vi "HIOKI PW3390 Acquisition Harmonic.vi"() -> ()   [LabVIEW 2009]
doc: "Outputs the harmonic measurement data and plots on a bar graph in 100ms cycle."
uses:
  <instrlib>/PW3390/Common/_Initialize/HIOKI PW3390 Initialize LAN.vi
  <instrlib>/PW3390/Common/_Initialize/HIOKI PW3390 Initialize RS-232C.vi
panel:
  out "error out":errorcluster
  in  "Communication Interface":enum16{"LAN", "RS-232C"}(ring)
  in  "COM Port":refnum<visa-resource-name>="COM1"
  in  "baud rate (38400bps)":u32=38400
  in  "IP Address":string="192.168.1.1"
  out "HP Phase":dbl[](graph)
  out "HI Phase":dbl[](graph)
  out "HU Phase":dbl[](graph)
  out "HP %":dbl[](graph)
  out "HI %":dbl[](graph)
  out "HU %":dbl[](graph)
  out "HU Value":dbl[](graph)
  out "HP Value":dbl[](graph)
  out "HI Value":dbl[](graph)
  out "Data out":dbl[](array[numeric])
  out "Selected Item out":string[](array[string])
  in  "Stop":bool
  in  "CH Select":T1(ring)
  # "Note:\n Please set configuration before starting the program.\nChanging configuration during running the program is invalid."
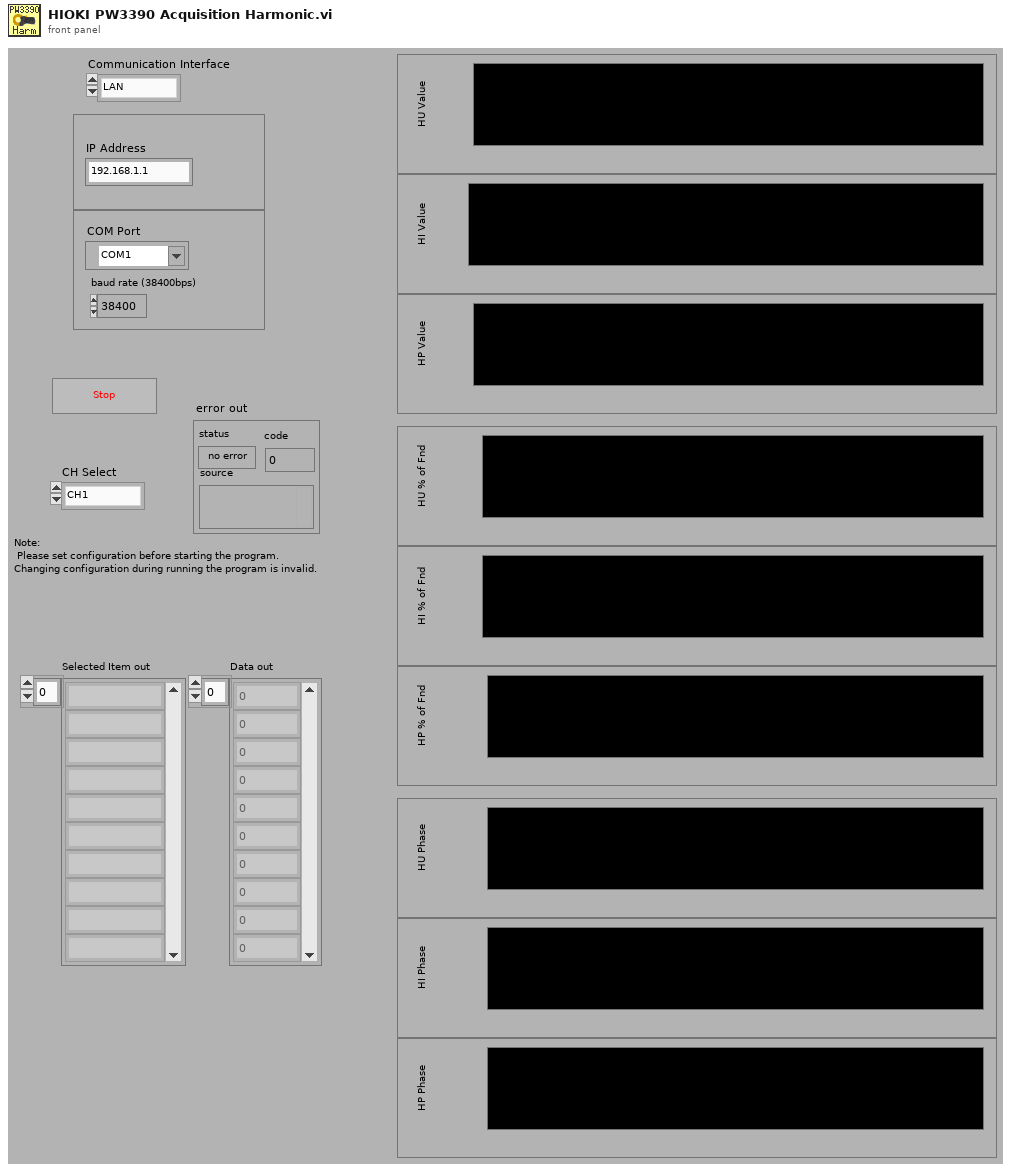
[diagram p1: front panel]
types:
  T1 = enum16{"CH1", "CH2", "CH3", "CH4", "CH12", "CH34", "CH123"}
  T2 = cluster{"LIST1":bool[], "LIST2":bool[], "LIST1 2":bool[], "LIST2 2":bool[], "LIST1 3":bool[], "LIST2 3":bool[]}
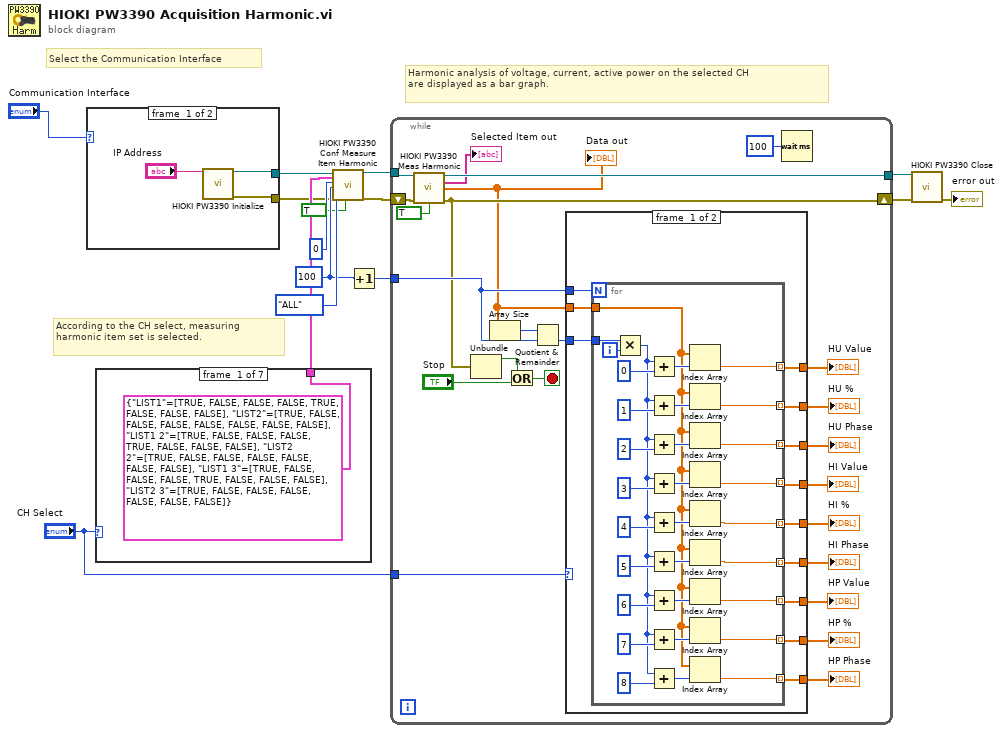
[diagram p0: block diagram]
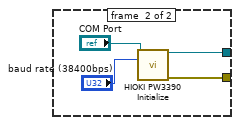
[diagram p2: hidden frame]
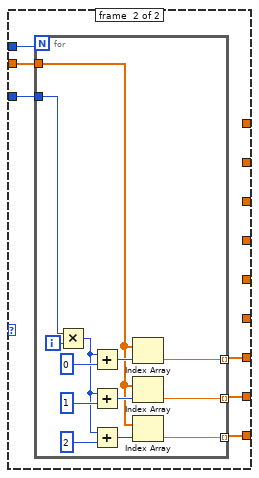
[diagram p3: hidden frame]
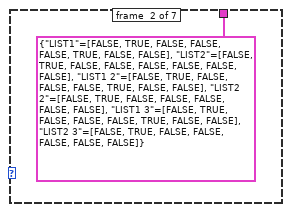
[diagram p4: hidden frame]
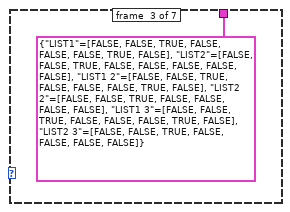
[diagram p5: hidden frame]
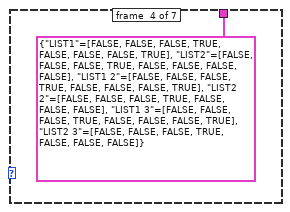
[diagram p6: hidden frame]
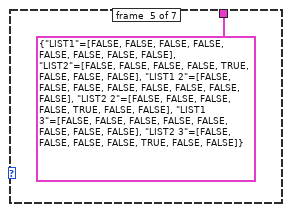
[diagram p7: hidden frame]
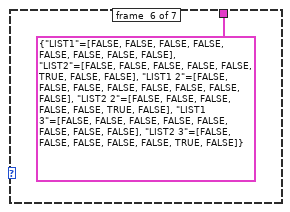
[diagram p8: hidden frame]
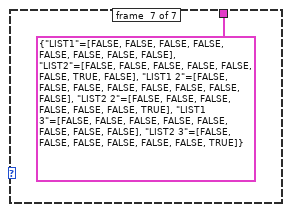
[diagram p9: hidden frame]
diagram:
  w7 = 100 ("Max order (100)")
  # "Select the Communication Interface"
  # "Harmonic analysis of voltage, current, active power on the selected CH \nare displayed as a bar graph."
  # "According to the CH select, measuring \nharmonic item set is selected."
  n1 = case shown="\"LAN\", デフォルト" "Communication Interface" {
    tunnel: [w17 w22] -> w4
    tunnel: [w16 w21] -> w3
    frame #0 {
      n2 = call-poly <instrlib>:"HIOKI PW3390 Initialize.vi"("IP Address"="IP Address") -> ("VISA Resource out"=w17:refnum<visa-resource-name>, "error out"=w16:errorcluster)  [unwired: 12 in, 1 out]
    }
    frame #1 {
      n3 = call-poly <instrlib>:"HIOKI PW3390 Initialize.vi"("COM Port"="COM Port", "baud rate (38400bps)"="baud rate (38400bps)") -> ("VISA Resource out"=w22:refnum<visa-resource-name>, "error out"=w21:errorcluster)  [unwired: 11 in, 1 out]
    }
  }
  n4 = case shown="\"CH4\"" "CH Select" {
    tunnel: [T2 {"LIST1"=[TRUE, FALSE, FALSE, FALSE, TRUE, FALSE, FALSE, FALSE], "LIST2"=[TRUE, FALSE, FALSE, FALSE, FALSE, FALSE, FALSE, FALSE], "LIST1 2"=[TRUE, FALSE, FALSE, FALSE, TRUE, FALSE, FALSE, FALSE], "LIST2 2"=[TRUE, FALSE, FALSE, FALSE, FALSE, FALSE, FALSE], "LIST1 3"=[TRUE, FALSE, FALSE, FALSE, TRUE, FALSE, FALSE, FALSE], "LIST2 3"=[TRUE, FALSE, FALSE, FALSE, FALSE, FALSE, FALSE]} ("LIST") T2 {"LIST1"=[FALSE, TRUE, FALSE, FALSE, FALSE, TRUE, FALSE, FALSE], "LIST2"=[FALSE, TRUE, FALSE, FALSE, FALSE, FALSE, FALSE, FALSE], "LIST1 2"=[FALSE, TRUE, FALSE, FALSE, FALSE, TRUE, FALSE, FALSE], "LIST2 2"=[FALSE, TRUE, FALSE, FALSE, FALSE, FALSE, FALSE], "LIST1 3"=[FALSE, TRUE, FALSE, FALSE, FALSE, TRUE, FALSE, FALSE], "LIST2 3"=[FALSE, TRUE, FALSE, FALSE, FALSE, FALSE, FALSE]} ("LIST") T2 {"LIST1"=[FALSE, FALSE, TRUE, FALSE, FALSE, FALSE, TRUE, FALSE], "LIST2"=[FALSE, FALSE, TRUE, FALSE, FALSE, FALSE, FALSE, FALSE], "LIST1 2"=[FALSE, FALSE, TRUE, FALSE, FALSE, FALSE, TRUE, FALSE], "LIST2 2"=[FALSE, FALSE, TRUE, FALSE, FALSE, FALSE, FALSE], "LIST1 3"=[FALSE, FALSE, TRUE, FALSE, FALSE, FALSE, TRUE, FALSE], "LIST2 3"=[FALSE, FALSE, TRUE, FALSE, FALSE, FALSE, FALSE]} ("LIST") T2 {"LIST1"=[FALSE, FALSE, FALSE, TRUE, FALSE, FALSE, FALSE, TRUE], "LIST2"=[FALSE, FALSE, FALSE, TRUE, FALSE, FALSE, FALSE, FALSE], "LIST1 2"=[FALSE, FALSE, FALSE, TRUE, FALSE, FALSE, FALSE, TRUE], "LIST2 2"=[FALSE, FALSE, FALSE, TRUE, FALSE, FALSE, FALSE], "LIST1 3"=[FALSE, FALSE, FALSE, TRUE, FALSE, FALSE, FALSE, TRUE], "LIST2 3"=[FALSE, FALSE, FALSE, TRUE, FALSE, FALSE, FALSE]} ("LIST") T2 {"LIST1"=[FALSE, FALSE, FALSE, FALSE, FALSE, FALSE, FALSE, FALSE], "LIST2"=[FALSE, FALSE, FALSE, FALSE, TRUE, FALSE, FALSE, FALSE], "LIST1 2"=[FALSE, FALSE, FALSE, FALSE, FALSE, FALSE, FALSE, FALSE], "LIST2 2"=[FALSE, FALSE, FALSE, FALSE, TRUE, FALSE, FALSE], "LIST1 3"=[FALSE, FALSE, FALSE, FALSE, FALSE, FALSE, FALSE, FALSE], "LIST2 3"=[FALSE, FALSE, FALSE, FALSE, TRUE, FALSE, FALSE]} ("LIST") T2 {"LIST1"=[FALSE, FALSE, FALSE, FALSE, FALSE, FALSE, FALSE, FALSE], "LIST2"=[FALSE, FALSE, FALSE, FALSE, FALSE, TRUE, FALSE, FALSE], "LIST1 2"=[FALSE, FALSE, FALSE, FALSE, FALSE, FALSE, FALSE, FALSE], "LIST2 2"=[FALSE, FALSE, FALSE, FALSE, FALSE, TRUE, FALSE], "LIST1 3"=[FALSE, FALSE, FALSE, FALSE, FALSE, FALSE, FALSE, FALSE], "LIST2 3"=[FALSE, FALSE, FALSE, FALSE, FALSE, TRUE, FALSE]} ("LIST") T2 {"LIST1"=[FALSE, FALSE, FALSE, FALSE, FALSE, FALSE, FALSE, FALSE], "LIST2"=[FALSE, FALSE, FALSE, FALSE, FALSE, FALSE, TRUE, FALSE], "LIST1 2"=[FALSE, FALSE, FALSE, FALSE, FALSE, FALSE, FALSE, FALSE], "LIST2 2"=[FALSE, FALSE, FALSE, FALSE, FALSE, FALSE, TRUE], "LIST1 3"=[FALSE, FALSE, FALSE, FALSE, FALSE, FALSE, FALSE, FALSE], "LIST2 3"=[FALSE, FALSE, FALSE, FALSE, FALSE, FALSE, TRUE]} ("LIST")] -> w15
    frame #0 {
    }
    frame #1 {
    }
    frame #2 {
    }
    frame #3 {
    }
    frame #4 {
    }
    frame #5 {
    }
    frame #6 {
    }
  }
  n5 = call <instrlib>:"HIOKI PW3390 Conf Measure Item Harmonic.vi"("VISA Resource"=w4, "LIST"=w15, "Min Order (0)"=0 ("Min order (0)"), "Max Order (100)"=w7, "ODD/EVEN/ALL (2: ALL)"=enum16{"ODD", "EVEN", "ALL"}."ALL", "error in (no error)"=w3, "Error Out (F: Off)"=TRUE) -> ("VISA Resource out"=w11:refnum<visa-resource-name>, "error out"=w10:errorcluster)  [unwired: 7 in, 4 out]
  n6 = Increment(x=w7) -> (x+1=w14:i32)
  n7 = while {
    tunnel: [w44] -> w9
    shift-right: [w46] -> w8
    shift-left: w10 -> [w45]
    tunnel: w14 -> [w49]
    tunnel: w11 -> [w41]
    tunnel: "CH Select" -> [w40]
    stop <- w53 stop-if-true
    n8 = call <instrlib>:"HIOKI PW3390 Meas Harmonic.vi"("VISA Resource"=w41, "error in (no error)"=w45, "Error Out (F: Off)"=TRUE) -> ("VISA Resource out"=w44:refnum<visa-resource-name>, "Selected Item out"=→"Selected Item out":string[], "Data out"=w43:dbl[], "error out"=w46:errorcluster)  [unwired: 7 in, 2 out]
    "Data out" <- w43
    n9 = Unbundle(w46) -> ("status"=w51:bool)  [unwired: 2 out]
    n10 = Array Size(array=w43) -> (size(s)=w47:i32)
    n11 = Or(x=w51, y="Stop") -> (x .or. y?=w53:bool)
    n12 = Quotient & Remainder(x=w47, y=w49) -> (floor(x/y)=w48:i32)  [unwired: 1 out]
    n13 = case shown="\"CH12\".." w40 {
      tunnel: w49 -> [w65 w97]
      tunnel: w48 -> [w64 w101]
      tunnel: w43 -> [w63 w102]
      tunnel: [w62 _] -> w39
      tunnel: [w61 _] -> w38
      tunnel: [w60 _] -> w37
      tunnel: [w59 _] -> w36
      tunnel: [w58 _] -> w35
      tunnel: [w57 _] -> w34
      tunnel: [w56 w99] -> w33
      tunnel: [w55 w100] -> w32
      tunnel: [w54 w98] -> w31
      frame #0 {
        n14 = for {
          N: w65 -> [_]
          tunnel: w63 -> [w74]
          tunnel: w64 -> [w96]
          tunnel: [w68] -> w62 mode=indexing
          tunnel: [w91] -> w61 mode=indexing
          tunnel: [w90] -> w60 mode=indexing
          tunnel: [w67] -> w59 mode=indexing
          tunnel: [w73] -> w58 mode=indexing
          tunnel: [w72] -> w57 mode=indexing
          tunnel: [w66] -> w56 mode=indexing
          tunnel: [w71] -> w55 mode=indexing
          tunnel: [w70] -> w54 mode=indexing
          i -> [w95]
          n15 = Multiply(x=w96, y=w95) -> (x*y=w69:i32)
          n16 = Add(x=w69, y=0) -> (x+y=w94:i32)
          n17 = Add(x=w69, y=1) -> (x+y=w93:i32)
          n18 = Add(x=w69, y=2) -> (x+y=w92:i32)
          n19 = Add(x=w69, y=3) -> (x+y=w85:i32)
          n20 = Add(x=w69, y=4) -> (x+y=w84:i32)
          n21 = Add(x=w69, y=5) -> (x+y=w81:i32)
          n22 = Add(x=w69, y=6) -> (x+y=w80:i32)
          n23 = Add(x=w69, y=7) -> (x+y=w77:i32)
          n24 = Add(x=w69, y=8) -> (x+y=w76:i32)
          n25 = Index Array(array=w74, index=w94) -> (element=w68:dbl)
          n26 = Index Array(array=w74, index=w93) -> (element=w91:dbl)
          n27 = Index Array(array=w74, index=w92) -> (element=w90:dbl)
          n28 = Index Array(array=w74, index=w85) -> (element=w67:dbl)
          n29 = Index Array(array=w74, index=w84) -> (element=w73:dbl)
          n30 = Index Array(array=w74, index=w81) -> (element=w72:dbl)
          n31 = Index Array(array=w74, index=w80) -> (element=w66:dbl)
          n32 = Index Array(array=w74, index=w77) -> (element=w71:dbl)
          n33 = Index Array(array=w74, index=w76) -> (element=w70:dbl)
        }
      }
      frame #1 {
        n34 = for {
          N: w97 -> [_]
          tunnel: w102 -> [w105]
          tunnel: w101 -> [w115]
          tunnel: [w103] -> w99 mode=indexing
          tunnel: [w110] -> w100 mode=indexing
          tunnel: [w109] -> w98 mode=indexing
          i -> [w114]
          n35 = Multiply(x=w115, y=w114) -> (x*y=w104:i32)
          n36 = Add(x=w104, y=0) -> (x+y=w113:i32)
          n37 = Add(x=w104, y=1) -> (x+y=w112:i32)
          n38 = Add(x=w104, y=2) -> (x+y=w111:i32)
          n39 = Index Array(array=w105, index=w113) -> (element=w103:dbl)
          n40 = Index Array(array=w105, index=w112) -> (element=w110:dbl)
          n41 = Index Array(array=w105, index=w111) -> (element=w109:dbl)
        }
      }
    }
    "HP Phase" <- w31
    "HP %" <- w32
    "HP Value" <- w33
    "HI Phase" <- w34
    "HI %" <- w35
    "HI Value" <- w36
    "HU Phase" <- w37
    "HU %" <- w38
    "HU Value" <- w39
    n42 = Wait (ms)(milliseconds to wait=u32 100) -> ()  [unwired: 1 out]
  }
  n43 = call <instrlib>:"HIOKI PW3390 Close.vi"("VISA Resource"=w9, "error in (no error)"=w8) -> ("error out"=→"error out":errorcluster)  [unwired: 13 in]
